vi "Queue Mailbox Valid.vi"(11 "Base Queue jettl in":refnum<class "Base Queue jettl.lvclass">) -> (2 "Valid?":bool)   [LabVIEW 2021, in "jettl.lvlib" / "Base Queue jettl.lvlib" / "Base Queue jettl.lvclass"]
uses:
  Base Queue jettl.lvclass
  Base Queue jettl.lvclass/Base Queue jettl.ctl
  Queue Mailbox/Queue Mailbox.lvclass
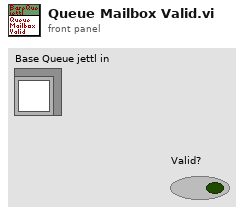
[diagram p1: front panel]
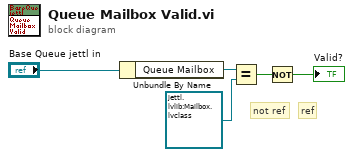
[diagram p0: block diagram]
diagram:
  # "ref"
  # "not ref"
  n1 = Unbundle By Name("Base Queue jettl in") -> ("Queue Mailbox"=w4:refnum<data-value>)
  n2 = Equal?(x=w4, y=refnum<data-value> refnum ("Queue Mailbox")) -> (x = y?=w2:bool)
  n3 = Not(x=w2) -> (.not. x?=→"Valid?":bool)
